vi "UI_AutoRefresh_Do.vi"(8 "error in (no error)":errorcluster, 9 "Parameters":T1={"Write TipStrips with details (T)"=TRUE, "Write Captions with UserLabels (T)"=TRUE, "Mode (ind only)"=enum."Indicators only", "Enable nested stream (T)"=TRUE}, 10 "Databox_sealed":refnum<class "Databox_sealed.lvclass">, 11 "SCHEMA_03 in":refnum<class "SCHEMA_03.lvclass">) -> (0 "error out":errorcluster, 3 "SCHEMA_03 out":refnum<class "SCHEMA_03.lvclass">)   [LabVIEW 2020, in "SCHEMA_03.lvlib" / "SCHEMA_03.lvclass"]
doc: "Enable nested stream : Permet le routage de la databox vers les nested UIA de l'acteur. On peut couper ce ruissellement si les nested n'ont pas besoin de databox pour optimiser le programme."
uses:
  SCHEMA_03.lvclass
  D:/Projets/STEP AT/LUGE 2022.2/UIA_Demo/support/UI_Actor.lvlibp/UI_Actor/UI_Actor.lvclass
  support/UI_Actor.lvlibp/UI_Actor/ctl_AR_Parameters.ctl
  support/UI_Actor.lvlibp/UI_Actor/ctl_AR_Mode.ctl
  support/Databox.lvlibp/Databox_sealed/Databox_sealed.lvclass
  D&C_SchemaBase/D&C_SchemaBase/D&C_SchemaBase.lvclass
  support/UI_Actor.lvlibp/UI_Actor/UI_Elmt_Ref(Label).vi
  support/UI_Actor.lvlibp/UI_Actor/UI_Actor.lvclass
  D:/Projets/STEP AT/LUGE 2022.2/UIA_Demo/D&Cs/D&C_SchemaBase/D&C_SchemaBase/D&C_SchemaBase.lvclass
  D:/Projets/STEP AT/LUGE 2022.2/UIA_Demo/support/Actor Framework.lvlibp/1abvi3w/vi.lib/ActorFramework/Actor/Actor.lvclass
  D:/Projets/STEP AT/LUGE 2022.2/UIA_Demo/D&Cs/SCHEMA_03/SCHEMA_03/SCHEMA_03.lvclass
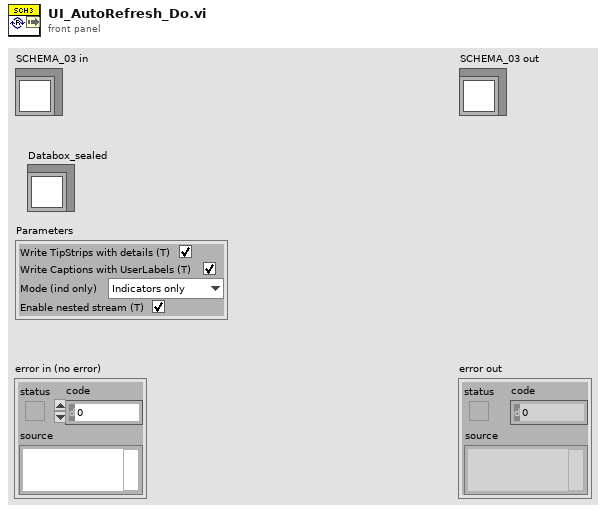
[diagram p1: front panel]
types:
  T1 = typedef "UI_Actor.lvlibp/UI_Actor.lvclass/ctl_AR_Parameters.ctl" = cluster{"Write TipStrips with details (T)":bool, "Write Captions with UserLabels (T)":bool, "Mode (ind only)":T2, "Enable nested stream (T)":bool}
  T2 = typedef "UI_Actor.lvlibp/UI_Actor.lvclass/ctl_AR_Mode.ctl" = enum16{"Controls only", "Indicators only", "All"}
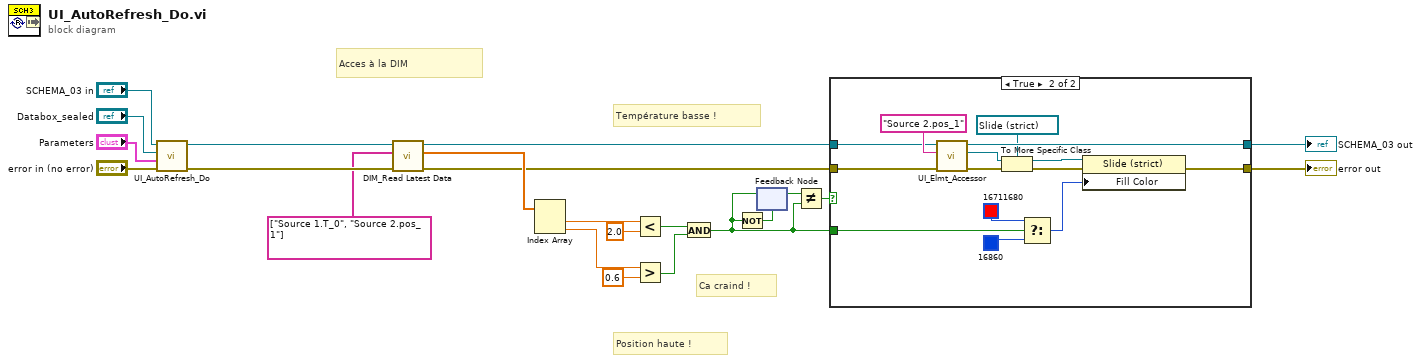
[diagram p0: block diagram]
diagram:
  # "Acces à la DIM"
  # "Ca craind !"
  # "Position haute !"
  # "Température basse !"
  n1 = call-parent "UI_AutoRefresh_Do.vi"("error in (no error)"="error in (no error)", "Parameters"="Parameters", "Databox_sealed"="Databox_sealed", "UI_Actor in"="SCHEMA_03 in") -> ("error out"=w17:errorcluster, "UI_Actor out"=w18:refnum<class "SCHEMA_03.lvclass">)  [unwired: 6 in]
  n2 = call "DIM_Read Latest Data.vi"("error in (no error)"=w17, "Src.SysLabels"=string[] ["Source 1.T_0", "Source 2.pos_1"], "UI_Actor in"=w18) -> ("error out"=w8:errorcluster, "Latest Data"=w15:dbl[], "UI_Actor out"=w7:refnum<class "SCHEMA_03.lvclass">)  [unwired: 6 in]
  n3 = Index Array(array=w15) -> (element #1=w14:dbl, element #2=w12:dbl)  [unwired: 2 in]
  n4 = Less?(x=w14, y=2.0) -> (x < y?=w10:bool)
  n5 = Greater?(x=w12, y=0.6) -> (0:w9:bool)
  n6 = And(x=w10, y=w9) -> (x .and. y?=w3:bool)
  n7 = Not(x=w3) -> (.not. x?=w2:bool)
  n8 = feedback-in #1(w3) -> ()
  n9 = feedback #1(w2) -> (w4:bool)
  n10 = Not Equal?(x=w4, y=w3) -> (x != y?=w1:bool)
  n11 = case shown="True" w1 {
    tunnel: w8 -> [w23 w37]
    tunnel: w7 -> [w24 w36]
    tunnel: [w24 w35] -> w6
    tunnel: [w23 w33] -> w5
    tunnel: w3 -> [_ w25]
    frame False {
    }
    frame True {
      n12 = call-poly "UI_Elmt_Accessor.vi"("error in (no error)"=w37, "Elmt Label"="Source 2.pos_1" ("SysLabel"), "UI_Actor in"=w36) -> ("error out"=w31:errorcluster, "Ctl Refnum"=w34:refnum<vi>, "UI_Actor out"=w35:refnum<class "SCHEMA_03.lvclass">)  [unwired: 5 in, 1 out]
      n13 = To More Specific Class(target class=refnum<vi> refnum ("Source 2.pos_1"), reference=w34, error in=w31) -> (specific class reference=w32:refnum<vi>, error out=w30:errorcluster)
      n14 = Select(t=u32 16711680, s=w25, f=u32 16860) -> (s? t:f=w26:u32)
      n15 = property class="Slide (strict)"(reference=w32, error in=w30, "Fill Color"=w26) -> (error out=w33:errorcluster)  [unwired: 1 out]
    }
  }
  "error out" <- w5
  "SCHEMA_03 out" <- w6
